vi "simpleCounterQH.vi"(8 "CounterEntry":u32, 10 "whichPMT?":u8 format="%08b") -> (0 "SPCtrWriteTimeout":bool)   [LabVIEW 2014]
uses:
  <vilib>/rvi/Emulation/niFpgaSctlEmulationGetInTimedLoop.vi
  <vilib>/rvi/interface/RandomDataEmulation/niFpgaRandomDataHandleErrors.vi
  queueHandlerGlobals.vi
  <vilib>/rvi/Emulation/niFpgaProcessEmulError.vi
  <vilib>/rvi/DataTransferAndStorage/Container/XNode/niFpgaContainer.xnode
  <vilib>/rvi/interface/RandomDataEmulation/nirviRandomDataFpgaReadWriteTemplate.vi
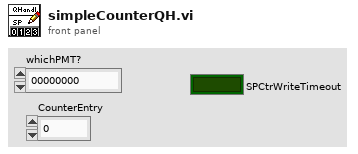
[diagram p1: front panel]
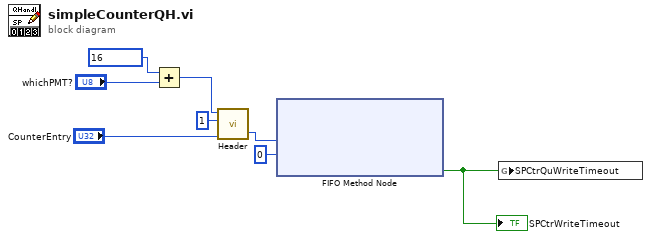
[diagram p0: block diagram]
diagram:
  n1 = Add(x=u8 16, y="whichPMT?") -> (x+y=w6:u8)
  n2 = call "Header.vi"("23BitData"="CounterEntry", "1BitHeaderIndex"=u8 1, "8BitHead"=w6) -> ("32BitOutput"=w4:u32)  [unwired: 2 in]
  n3 = xnode ("FIFO Method Node")("Element"=w4, "Timeout"=0) -> ("Timed Out?"=w2:bool)  [unwired: 1 in, 1 out]
  "SPCtrWriteTimeout" <- w2
  n4 = global write "queueHandlerGlobals.vi" "SPCtrQuWriteTimeout"(w2) -> ()
